vi "comm get user string.vi"(8 "error in (no error)":errorcluster, 11 "Comm Handle":u32) -> (0 "error out":errorcluster, 2 "user string":string, 3 "dup Comm Handle":u32)   [LabVIEW 2013, in "lvserial.lvlib"]
doc: "Retrieves the user string. The user string is private data value and is unique per serial port. This value is not used by the serial port library for any purpose."
uses:
  lvserial.lvlib
  lvserial.dll
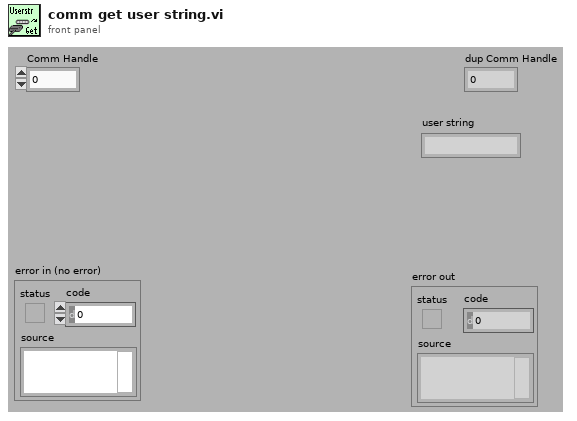
[diagram p1: front panel]
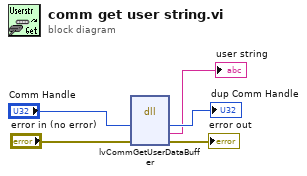
[diagram p0: block diagram]
diagram:
  n1 = dll-call lib="lvserial.dll" fn="lvCommGetUserDataBuffer"("hComm"="Comm Handle", "error in (no error)"="error in (no error)") -> ("hComm"=→"dup Comm Handle":u32, "shUserData"=→"user string":string, "error in (no error)"=→"error out":errorcluster)  [unwired: 3 in, 4 out]
